vi "MA filter.vi"(1 "dt":dbl, 2 "Tw":dbl, 3 "y_1":dbl, 4 "y":dbl) -> (0 "yf":dbl)   [LabVIEW 2023]
panel:
  # "Out"
  # "In"
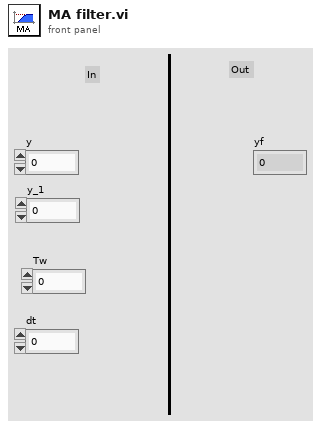
[diagram p1: front panel]
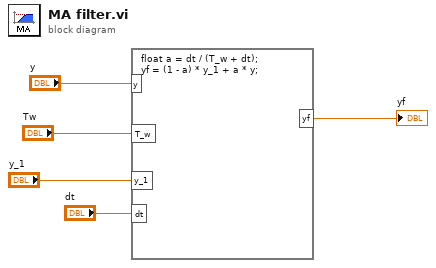
[diagram p0: block diagram]
diagram:
  n1 = formula code="float a = dt / (T_w + dt);\nyf = (1 - a) * y_1 + a * y;"("y"="y", "T_w"="Tw", "y_1"="y_1", "dt"="dt") -> ("yf"=→"yf":dbl)
